vi "Create Queue.vi"(9 "Queue jettl":refnum<class "Queue jettl.lvclass">, 10 "Alias":string, 11 "Create Queue in":refnum<class "Create Queue.lvclass">) -> (3 "Create Queue out":refnum<class "Create Queue.lvclass">)   [LabVIEW 2021, in "jettl Msg Create Queue.lvlib" / "Create Queue.lvclass"]
uses:
  Create Queue.lvclass
  jettl/Queue jettl/Queue jettl.lvclass
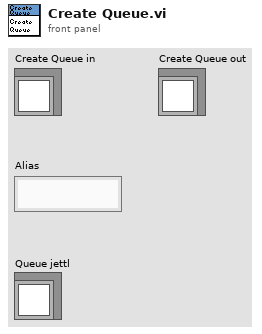
[diagram p1: front panel]
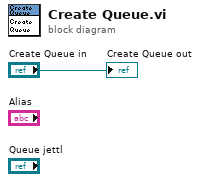
[diagram p0: block diagram]
diagram:
  "Create Queue out" <- "Create Queue in"
